vi "Nand.vi"(4 "b":bool, 5 "a":bool) -> (1 "out":bool)   [LabVIEW 2014]
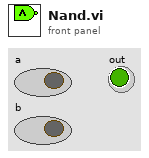
[diagram p1: front panel]
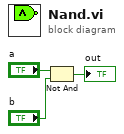
[diagram p0: block diagram]
diagram:
  n1 = Not And(1:"b", 2:"a") -> (0:→"out":bool)
